vi "RESET SWITCH.vi"() -> ()   [LabVIEW 2017]
panel:
  in  "Array 2":string[](array[string])=["192.168.10.20", "192.168.10.22"]
  in  "SMA mode":bool=TRUE
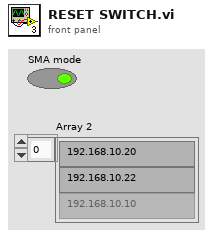
[diagram p1: front panel]
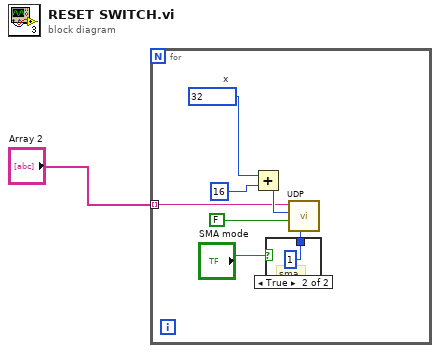
[diagram p0: block diagram]
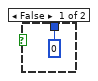
[diagram p2: hidden frame]
diagram:
  n1 = for {
    tunnel: "Array 2" -> [w2] mode=indexing
    w4 = u16 32  # x
    n2 = Add(x=w4, y=u32 16 ("Address")) -> (x+y=w3:u32)
    n3 = case shown="True" "SMA mode" {
      tunnel: [u8 0 ("In") u8 1 ("In")] -> w7
      frame False {
      }
      frame True {
        # "sma"
      }
    }
    n4 = call "UDP.vi"("In"=w7, "Read (TRUE)"=FALSE, "Address"=w3, "IP address"=w2) -> ()  [unwired: 5 in, 2 out]
  }
